vi "Read Streaming Peaks and Levels.vi"(8 "error in (no error)":errorcluster, 11 "VISA resource name":refnum<visa-resource-name>) -> (0 "error out":errorcluster, 1 "Peak Wavelengths (nm)":dbl[][](array[numeric]) format="%#_10g", 2 "Number of Sensors":u16[](array[numeric]), 3 "VISA resource name out":refnum<visa-resource-name>, 5 "Data Status":T1 {"Sub-Channel" items=["None", "1", "2", "3", "4"]; "Time Stamp" format="%#_20f"})   [LabVIEW 2015, in "Micron Optics sm130.lvlib"]
doc: "Reads data from the instrument when it is in streaming mode. Does not write a command to the instrument since the command is generated internally during streaming mode."
uses:
  Micron Optics sm130.lvlib
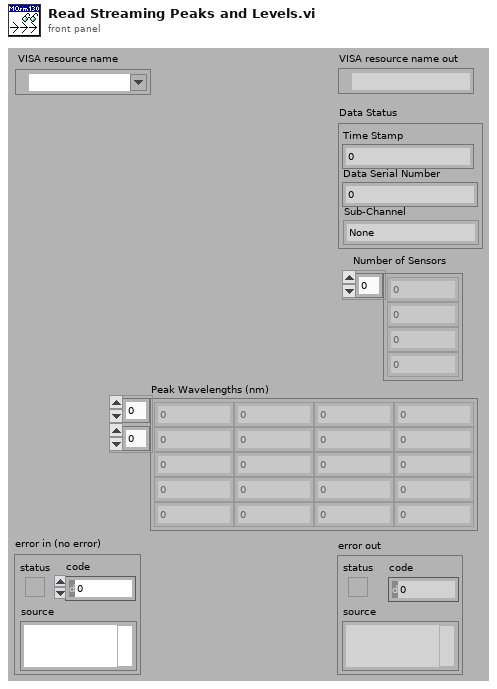
[diagram p1: front panel]
types:
  T1 = cluster{"Data Serial Number":u32, "Time Stamp":dbl, "Sub-Channel":u8}
  T2 = cluster{"Full Spectrum Radix":u8, "Firmware Version":u8, "Primary Fan":bool, "Secondary Fan":bool, "Switch Position":u8, "MUX":u8, "Trigger Mode":u8, "Operating Mode":u8, "Data Serial Number":u32, "Time Stamp":dbl, "Buffer (%)":u8, "MUX Level":u8}
  T3 = cluster{"Data Serial Number":u32, "Time Stamp":dbl, "Switch Position":u8}
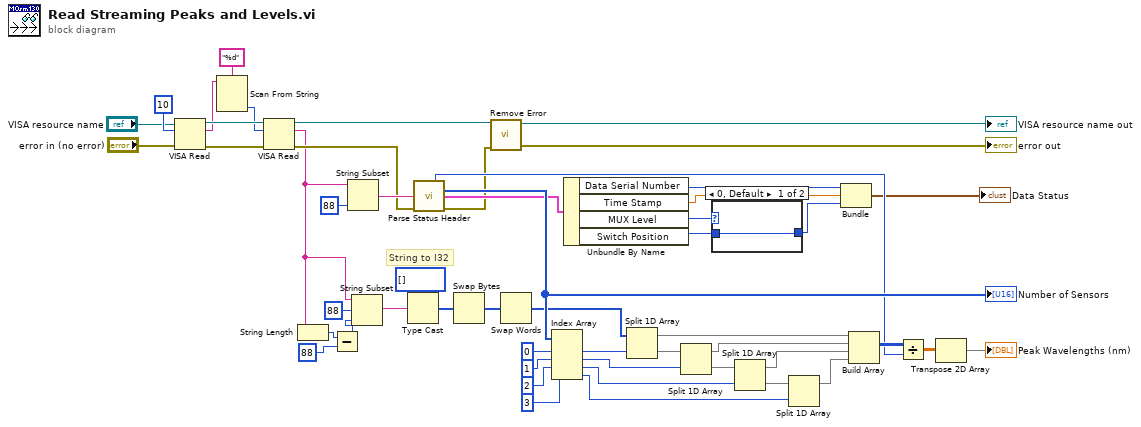
[diagram p0: block diagram]
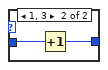
[diagram p2: hidden frame]
diagram:
  # "String to I32"
  n1 = VISA Read(VISA resource name="VISA resource name", byte count=u32 10, error in (no error)="error in (no error)") -> (VISA resource name out=w52:refnum<visa-resource-name>, read buffer=w49:string, error out=w51:errorcluster)  [unwired: 1 out]
  n2 = Scan From String(format string="%d", input string=w49) -> (output 1=w48:i32)  [unwired: 3 in, 3 out]
  n3 = VISA Read(VISA resource name=w52, byte count=w48, error in (no error)=w51) -> (VISA resource name out=w47:refnum<visa-resource-name>, read buffer=w3:string, error out=w9:errorcluster)  [unwired: 1 out]
  n4 = String Length(string=w3) -> (length=w6:i32)
  n5 = Subtract(x=w6, y=88) -> (x-y=w4:i32)
  n6 = String Subset(string=w3, length (rest)=88 ("length (rest)")) -> (substring=w43:string)  [unwired: 1 in]
  n7 = String Subset(string=w3, offset (0)=88 ("length (rest)"), length (rest)=w4) -> (substring=w36:string)
  n8 = Type Cast(type=i32[] [], x=w36) -> (*(type *) &x=w33:i32[])
  n9 = call "Parse Status Header.vi"("Status Header In"=w43, "error in (no error)"=w9) -> ("Granularity"=w23:u32, "Number of Sensors"=w41:u16[], "Status"=w16:T2, "error out"=w8:errorcluster)  [unwired: 7 in, 3 out]
  "Number of Sensors" <- w41
  n10 = Swap Bytes(anything=w33) -> (byte swapped=w34:i32[])
  n11 = call "Remove Error.vi"("error in (no error)"=w8, "VISA resource name"=w47) -> ("error out"=→"error out":errorcluster, "VISA resource name out"=→"VISA resource name out":refnum<visa-resource-name>)  [unwired: 8 in]
  n12 = Swap Words(1:w34) -> (0:w32:i32[])
  n13 = Index Array(array=w41, index #1=0 ("index"), index #2=1 ("index"), index #3=2 ("index"), index #4=3 ("index")) -> (element #1=w20:u16, element #2=w19:u16, element #3=w18:u16, element #4=w17:u16)
  n14 = Unbundle By Name(w16) -> ("Data Serial Number"=w15:u32, "Time Stamp"=w14:dbl, "MUX Level"=w12:u8, "Switch Position"=w11:u8)
  n15 = Split 1D Array(array=w32, index=w20) -> (first subarray=w28:i32[], second subarray=w31:i32[])
  n16 = Split 1D Array(array=w31, index=w19) -> (first subarray=w27:i32[], second subarray=w30:i32[])
  n17 = case shown="0, Default" w12 {
    tunnel: w11 -> [w53 w55]
    tunnel: [w53 w54] -> w10
    frame 0, Default {
    }
    frame 1, 3 {
      n18 = Increment(x=w55) -> (x+1=w54:u8)
    }
  }
  n19 = Split 1D Array(array=w30, index=w18) -> (first subarray=w26:i32[], second subarray=w29:i32[])
  n20 = Split 1D Array(array=w29, index=w17) -> (first subarray=w25:i32[])  [unwired: 1 out]
  n21 = Bundle("Data Serial Number"=w15, "Time Stamp"=w14, "Switch Position"=w10) -> (→"Data Status":T3)  [unwired: 1 in]
  n22 = Build Array(w28, w27, w26, w25) -> (w24:i32[][])
  n23 = Divide(x=w24, y=w23) -> (x/y=w22:dbl[][])
  n24 = Transpose 2D Array(2D array=w22) -> (transposed array=→"Peak Wavelengths (nm)":dbl[][])
